vi "PmodACLRead.vi"(7 "I2C Channel (0)":u8, 8 "Error In":errorcluster, 9 "Resolution":enum16{"2g", "4g", "8g", "16g"}(ring), 10 "ADXL345 Address":T2, 11 "LINX Resource":T3) -> (0 "Error Out":errorcluster, 2 "Acceleration Data (g)":T1, 3 "LINX Resource":T3)   [LabVIEW 2014]
doc: "Read acceleration data (in g's) from the ADXL345."
uses:
  <vilib>/MakerHub/LINX/Private/Type Defs/LINX Ref.ctl
  <vilib>/MakerHub/LINX/Private/Type Defs/Platform.ctl
  <vilib>/MakerHub/LINX/Private/Type Defs/Interface.ctl
  <vilib>/MakerHub/LINX/Private/Device/Type Defs/LINX Device Config.ctl
  <vilib>/MakerHub/LINX/Private/Device/Type Defs/TCP Config.ctl
  <vilib>/MakerHub/LINX/Private/Device/Type Defs/Channels.ctl
  <vilib>/MakerHub/LINX/Public/Sensors/Accelerometer/ADXL345/Address.ctl
  <vilib>/MakerHub/LINX/LMH-LINX.lvlib
  <vilib>/MakerHub/Toolbox/LMH-Toolbox.lvlib
  <vilib>/MakerHub/LINX/Private/Device/Device.lvlib
  <vilib>/MakerHub/LINX/Public/Sensors/Accelerometer/ADXL345/ADXL345.lvlib
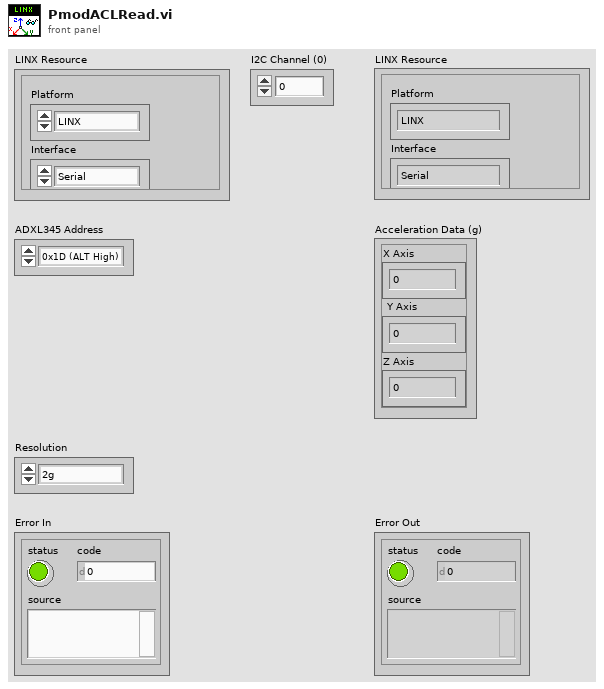
[diagram p1: front panel]
types:
  T1 = cluster{"X Axis":dbl, "Y Axis":dbl, "Z Axis":dbl}
  T2 = typedef "LMH-LINX.lvlib/ADXL345.lvlib/Address.ctl" = enum16{"0x1D (ALT High)", "0x53 (ALT Low)"}
  T3 = typedef "LMH-LINX.lvlib/LINX Ref.ctl" = cluster{"Platform":T4, "Interface":T5, "LINX Device Config":T6}
  T4 = typedef "LMH-LINX.lvlib/Platform.ctl" = enum16{"LINX", "myRIO"}
  T5 = typedef "LMH-LINX.lvlib/Interface.ctl" = enum16{"Serial", "TCP"}
  T6 = typedef "LMH-LINX.lvlib/Device.lvlib/LINX Device Config.ctl" = cluster{"Interface":T5, "COM Port":refnum<visa-resource-name>, "TCP Configuration":T7, "Device Family":u8, "Device ID":u8, "Device Name":string, "TCP Ref":refnum<k5>, "Channels":T8}
  T7 = typedef "LMH-LINX.lvlib/Device.lvlib/TCP Config.ctl" = cluster{"IP Address":string, "Port":u16}
  T8 = typedef "LMH-LINX.lvlib/Channels.ctl" = cluster{"DI":u8[], "DO":u8[], "AI":u8[], "AO":u8[], "PWM":u8[], "QE":u8[], "UART":u8[], "I2C 2":u8[], "SPI":u8[], "CAN":u8[], "Servo":u8[], "AI Ref (V)":dbl, "AO Ref (V)":dbl, "AO Resolution (Bits)":u8}
  T9 = cluster{"Decimal I16":i16, "Decimal I16":i16, "Decimal I16":i16}
  T10 = cluster{"Decimal I16":dbl, "Decimal I16":dbl, "Decimal I16":dbl}
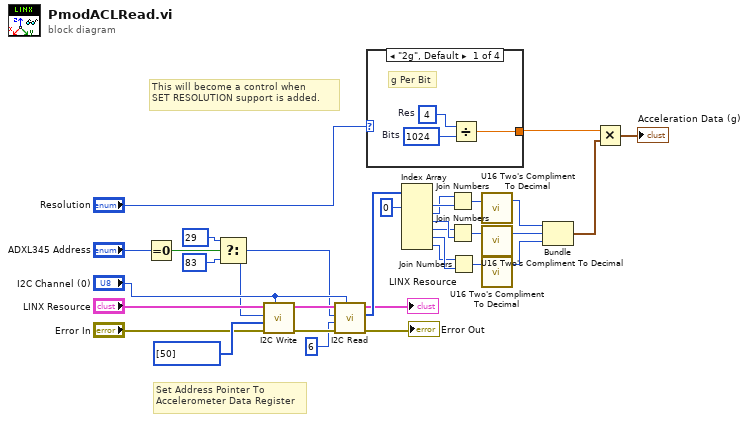
[diagram p0: block diagram]
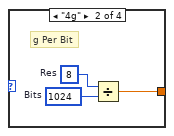
[diagram p2: hidden frame]
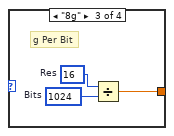
[diagram p3: hidden frame]
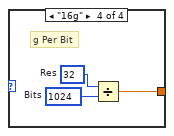
[diagram p4: hidden frame]
diagram:
  # "This will become a control when \nSET RESOLUTION support is added."
  # "Set Address Pointer To \nAccelerometer Data Register"
  n1 = Equal To 0?(x="ADXL345 Address") -> (x = 0?=w32:bool)
  n2 = Select(t=u8 29 ("I2C Slave Address (0)"), s=w32, f=u8 83 ("I2C Slave Address (0)")) -> (s? t:f=w3:u8)
  n3 = call <vilib>:"I2C Write.vi"("I2C Channel"="I2C Channel (0)", "Error In"="Error In", "Data"=u8[] [50], "I2C Slave Address (0)"=w3, "LINX Resource"="LINX Resource") -> ("Error Out"=w24:errorcluster, "LINX Resource"=w25:T3)  [unwired: 5 in]
  n4 = call <vilib>:"I2C Read.vi"("I2C Channel"="I2C Channel (0)", "Error In"=w24, "Bytes To Read"=u8 6, "I2C Slave Address (0)"=w3, "LINX Resource"=w25) -> ("Error Out"=→"Error Out":errorcluster, "Data"=w22:u8[], "LINX Resource"=→"LINX Resource":T3)  [unwired: 4 in]
  n5 = case shown="\"2g\", Default" "Resolution" {
    tunnel: [w33 w36 w39 w42] -> w8
    frame "2g", Default {
      w34 = 4  # Res
      w35 = 1024  # Bits
      # "g Per Bit"
      n6 = Divide(x=w34, y=w35) -> (x/y=w33:dbl)
    }
    frame "4g" {
      w37 = 8  # Res
      w38 = 1024  # Bits
      # "g Per Bit"
      n7 = Divide(x=w37, y=w38) -> (x/y=w36:dbl)
    }
    frame "8g" {
      w40 = 16  # Res
      w41 = 1024  # Bits
      # "g Per Bit"
      n8 = Divide(x=w40, y=w41) -> (x/y=w39:dbl)
    }
    frame "16g" {
      w43 = 32  # Res
      w44 = 1024  # Bits
      # "g Per Bit"
      n9 = Divide(x=w43, y=w44) -> (x/y=w42:dbl)
    }
  }
  n10 = Index Array(array=w22, index #1=0 ("index")) -> (element #1=w20:u8, element #2=w19:u8, element #3=w18:u8, element #4=w17:u8, element #5=w16:u8, element #6=w15:u8)  [unwired: 5 in]
  n11 = Join Numbers(hi=w19, lo=w20) -> ((hi.lo)=w14:u16)
  n12 = Join Numbers(hi=w17, lo=w18) -> ((hi.lo)=w13:u16)
  n13 = Join Numbers(hi=w15, lo=w16) -> ((hi.lo)=w12:u16)
  n14 = call <vilib>:"U16 Two's Compliment To Decimal.vi"("Two's Compliment U16"=w14) -> ("Decimal I16"=w11:i16)  [unwired: 2 in]
  n15 = call <vilib>:"U16 Two's Compliment To Decimal.vi"("Two's Compliment U16"=w13) -> ("Decimal I16"=w10:i16)  [unwired: 2 in]
  n16 = call <vilib>:"U16 Two's Compliment To Decimal.vi"("Two's Compliment U16"=w12) -> ("Decimal I16"=w9:i16)  [unwired: 2 in]
  n17 = Bundle("Decimal I16"=w11, "Decimal I16"=w10, "Decimal I16"=w9) -> (w7:T9)  [unwired: 1 in]
  n18 = Multiply(x=w8, y=w7) -> (x*y=→"Acceleration Data (g)":T10)
